vi "convertCompassRawDataToDeg.vi"(0 "raw x":sgl, 2 "offset":cluster{"x":sgl, "z":sgl, "y":sgl}, 3 "calc offset":bool, 7 "raw y":sgl, 11 "raw z":sgl) -> (4 "x":sgl, 8 "y":sgl, 14 "deg":sgl, 15 "z":sgl)   [LabVIEW 2025]
panel:
  in  "z scale [µT]":sgl=2500.0 format="%#_13g"
  in  "x,y scale [µT]":sgl=1300.0 format="%#_13g"
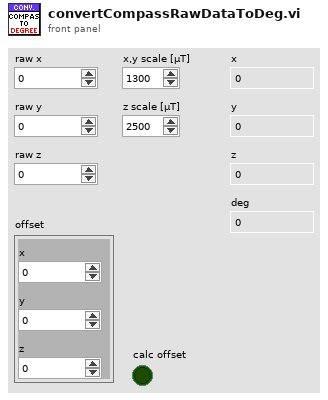
[diagram p1: front panel]
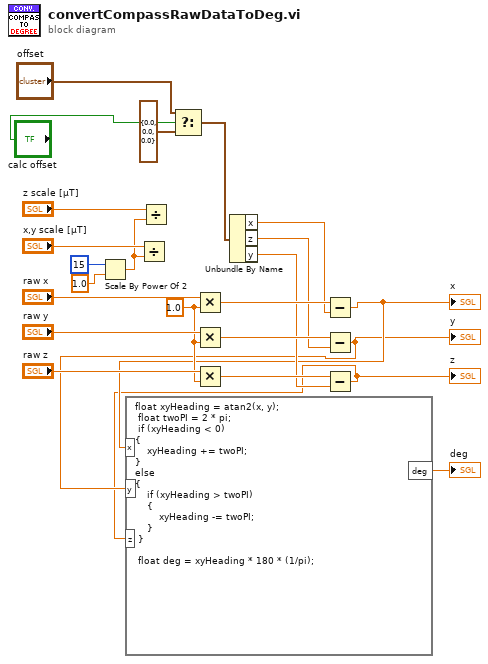
[diagram p0: block diagram]
diagram:
  w11 = sgl 1.0 ("y")
  n1 = Scale By Power Of 2(n=i16 15, x=sgl 1.0) -> (x*2^n=w16:sgl)
  n2 = Divide(x="x,y scale [µT]", y=w16) -> ()  [unwired: 1 out]
  n3 = Divide(x="z scale [µT]", y=w16) -> ()  [unwired: 1 out]
  n4 = Select(t="offset", s="calc offset", f=cluster{"x":sgl, "z":sgl, "y":sgl} {"x"=0.0, "z"=0.0, "y"=0.0}) -> (s? t:f=w5:cluster{"x":sgl, "z":sgl, "y":sgl})
  n5 = Multiply(x="raw x", y=w11) -> (x*y=w18:sgl)
  n6 = Multiply(x="raw y", y=w11) -> (x*y=w19:sgl)
  n7 = Multiply(x="raw z", y=w11) -> (x*y=w20:sgl)
  n8 = Unbundle By Name(w5) -> ("x"=w10:sgl, "z"=w9:sgl, "y"=w8:sgl)
  n9 = Subtract(x=w18, y=w10) -> (x-y=w3:sgl)
  "x" <- w3
  n10 = Subtract(x=w19, y=w9) -> (x-y=w2:sgl)
  "y" <- w2
  n11 = Subtract(x=w20, y=w8) -> (x-y=w1:sgl)
  "z" <- w1
  n12 = formula code="float xyHeading = atan2(x, y);\n\tfloat twoPI = 2 * pi;\n\tif (xyHeading < 0)\n{\n    xyHeading += twoPI;\n}\nelse \n{\n    if (xyHeading > twoPI) \n    { \n        xyHeading -= twoPI;\n    }\n\t}\n\t\n\tfloat deg = xyHeading * 180 * (1/pi);"("x"=w3, "y"=w2, "z"=w1) -> ("deg"=→"deg":dbl)
